vi "Check if Parameter Changed.vi"(8 "number of parameters":i32, 9 "first parameter index":i32, 10 "new values":dbl[](array[numeric]), 11 "previous values":dbl[](array[numeric])) -> (3 "parameter has changed":bool)   [LabVIEW 2020, in "AIM MIL-STD-1553 Engine.lvlib" / "Implementation.lvlib" / "Tx Execution Unit.lvclass"]
uses:
  Tx Execution Unit.lvclass
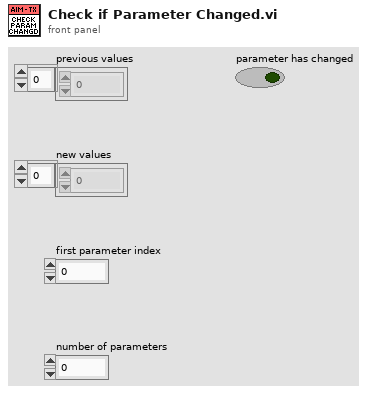
[diagram p1: front panel]
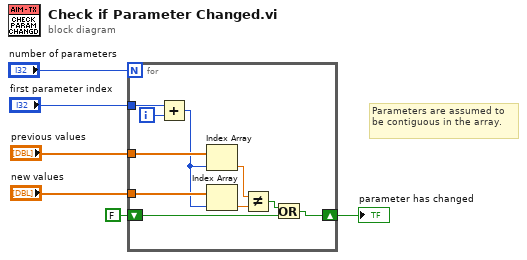
[diagram p0: block diagram]
diagram:
  # "Parameters are assumed to be contiguous in the array."
  n1 = for {
    N: "number of parameters" -> [_]
    tunnel: "first parameter index" -> [w9]
    tunnel: "previous values" -> [w15]
    tunnel: "new values" -> [w16]
    shift-right: [w11] -> w6
    shift-left: FALSE -> [w10]
    i -> [w7]
    n2 = Add(x=w9, y=w7) -> (x+y=w8:i32)
    n3 = Index Array(array=w15, index=w8) -> (element=w13:dbl)
    n4 = Index Array(array=w16, index=w8) -> (element=w14:dbl)
    n5 = Not Equal?(x=w13, y=w14) -> (x != y?=w12:bool)
    n6 = Or(x=w12, y=w10) -> (x .or. y?=w11:bool)
  }
  "parameter has changed" <- w6
